vi "_Get or Add Sheets.vi"(8 "error in":errorcluster, 10 "New Worksheetpart":refnum<k24>, 11 "Workbook in":refnum<k24>) -> (0 "error out":errorcluster, 2 "WorkbookPart":refnum<k24>, 3 "Workbook in out":refnum<k24>)   [LabVIEW 2021, in "Open Xml.lvlib"]
uses:
  Open Xml.lvlib
  D:/git/Open-Xml-LabVIEW/dll/DocumentFormat.OpenXml.dll
  dll/DocumentFormat.OpenXml.dll
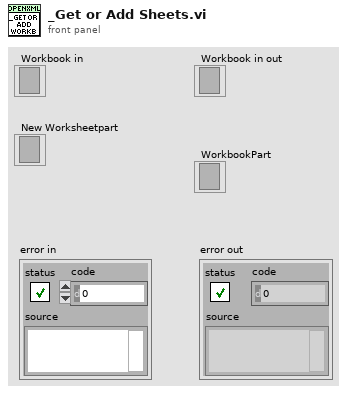
[diagram p1: front panel]
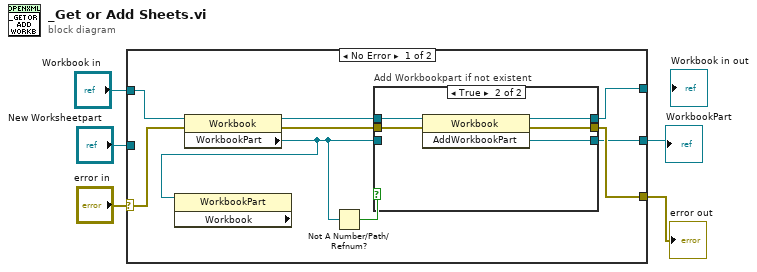
[diagram p0: block diagram]
diagram:
  n1 = case shown="No Error" "error in" {
    selector: "error in" -> [w15 w24]
    tunnel: [w9 w24] -> w5
    tunnel: "Workbook in" -> [w14 _]
    tunnel: [w10 _] -> w4
    tunnel: [w8 _] -> w3
    tunnel: "New Worksheetpart" -> [_ _]
    frame No Error {
      n2 = property class="Workbook"(reference=w14, error in=w15) -> (reference out=w12:refnum<k24>, error out=w11:errorcluster, "WorkbookPart"=w7:refnum<k24>)
      n3 = property class="WorkbookPart" props=["Workbook"](reference=w7) -> ()  [unwired: 1 in, 3 out]
      n4 = Not A Number/Path/Refnum?(number/path/refnum=w7) -> (NaN/Path/Refnum?=w13:bool)
      n5 = case "Add Workbookpart if not existent" shown="True" w13 {
        tunnel: w7 -> [w16 _]
        tunnel: w12 -> [w17 w23]
        tunnel: w11 -> [w18 w22]
        tunnel: [w17 w21] -> w10
        tunnel: [w18 w20] -> w9
        tunnel: [w16 w19] -> w8
        frame False {
        }
        frame True {
          n6 = invoke class="Workbook" method="AddWorkbookPart"(reference=w23, error in=w22) -> (reference out=w21:refnum<k24>, error out=w20:errorcluster, "AddWorkbookPart"=w19:refnum<k24>)  [unwired: 1 in]
        }
      }
    }
    frame Error {
    }
  }
  "error out" <- w5
  "WorkbookPart" <- w3
